vi "InitializeFpgaAcquisition.vi"(8 "error in (no error)":errorcluster, 11 "MCSA Acquisition Config":T1 {"FixedSizeX31"."InputConfig" items=["AC Coupled", "DC Coupled", "IEPE AC Coupled"]}) -> (0 "error out":errorcluster, 2 "start acquisition?":bool, 3 "dynamic FPGA VI reference":refnum<k20>)   [LabVIEW 2017, in "McsaFpgaAcquisition.lvlib"]
doc: "Initializes the acquisition of the dynamic channels with the RIO Wfm API."
uses:
  <vilib>/addons/InsightCM/Devices/Shared/Mcsa/McsaFpgaAcquisition/McsaFpgaAcquisition.lvlib
  <vilib>/addons/InsightCM/Devices/Shared/Mcsa/McsaFpgaAcquisition/controls/Configuration.ctl
  <vilib>/addons/InsightCM/Devices/Shared/Cms/CmsAcquisition/controls/FixedSizeArrays.ctl
  <vilib>/LabVIEW Targets/FPGA/cRIO/shared/nicrio_ModuleControls/nicrio_cRIO-9232_ConfigModeRing.ctl
  <vilib>/addons/InsightCM/Devices/Shared/Cms/cRIOWfmAcq/subVIs/RIO Wfm Cust Ctrls/rwfm_SamplingInfo.ctl
  <vilib>/addons/InsightCM/Devices/Shared/Mcsa/McsaFpgaAcquisition/controls/Group.ctl
  <vilib>/addons/InsightCM/Devices/Shared/Mcsa/McsaFpgaAcquisition/controls/ChannelMcsa.ctl
  <vilib>/addons/InsightCM/Devices/Shared/Mcsa/McsaFpgaAcquisition/controls/RangeParams.ctl
  <vilib>/Utility/error.llb/Error Cluster From Error Code.vi
  <vilib>/rvi/errors/niLvFpgaAdjustHostInterfaceError.vi
  <vilib>/rvi/interface/nirviReadWriteControl/nirviReadWriteControl.xnode
  <vilib>/addons/InsightCM/Devices/Shared/Mcsa/cRIOWfmAcqMcsa/cRIOWfmLibMcsa.lvlib
  NiFpgaLv.dll
  <vilib>/rvi/interface/Simulation/niFpgaSimulationCallBeginRW.vi
  <vilib>/addons/InsightCM/Devices/Shared/Cms/cRIOWfmAcq/cRIOWfmLib.lvlib
  <vilib>/addons/InsightCM/Devices/Shared/Cms/CmsAcquisition/CmsAcquisition.lvlib
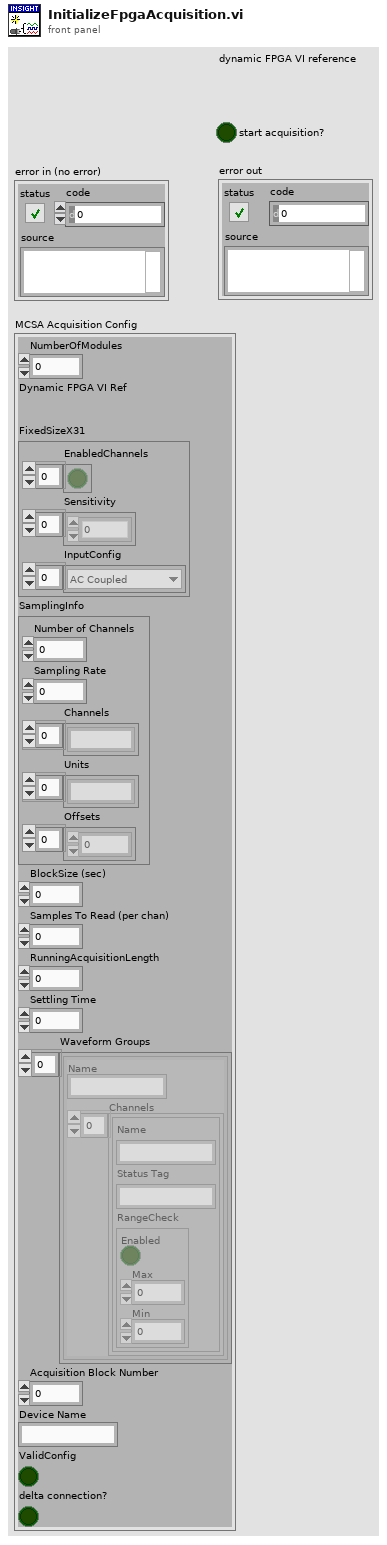
[diagram p1: front panel]
types:
  T1 = typedef "McsaFpgaAcquisition.lvlib/Configuration.ctl" = cluster{"NumberOfModules":i16, "Dynamic FPGA VI Ref":refnum<k20>, "FixedSizeX31":T2, "SamplingInfo":T4, "BlockSize (sec)":dbl, "Samples To Read (per chan)":i32, "RunningAcquisitionLength":dbl, "Settling Time":dbl, "Waveform Groups":T5[], "Acquisition Block Number":i32, "Device Name":string, "ValidConfig":bool, "delta connection?":bool}
  T2 = typedef "CmsAcquisition.lvlib/FixedSizeArrays.ctl" = cluster{"EnabledChannels":bool[], "Sensitivity":dbl[], "InputConfig":T3[]}
  T3 = typedef "nicrio_cRIO-9232_ConfigModeRing.ctl" = u8
  T4 = typedef "cRIOWfmLib.lvlib/rwfm_SamplingInfo.ctl" = cluster{"Number of Channels":i32, "Sampling Rate":dbl, "Channels":string[], "Units":string[], "Offsets":sgl[]}
  T5 = typedef "McsaFpgaAcquisition.lvlib/Group.ctl" = cluster{"Name":string, "Channels":T6[]}
  T6 = typedef "McsaFpgaAcquisition.lvlib/ChannelMcsa.ctl" = cluster{"Name":string, "Status Tag":string, "RangeCheck":T7}
  T7 = typedef "McsaFpgaAcquisition.lvlib/RangeParams.ctl" = cluster{"Enabled":bool, "Max":dbl, "Min":dbl}
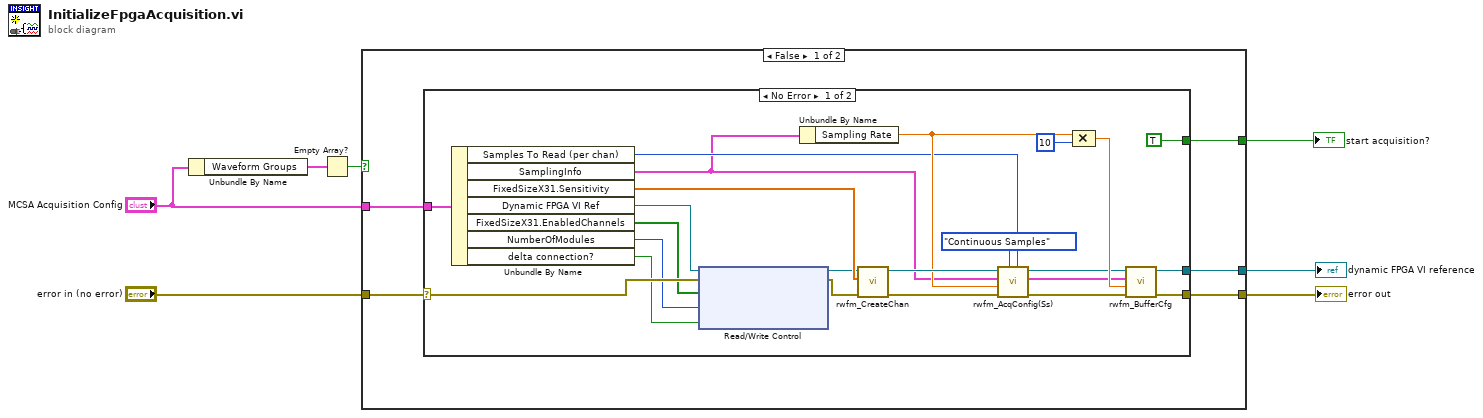
[diagram p0: block diagram]
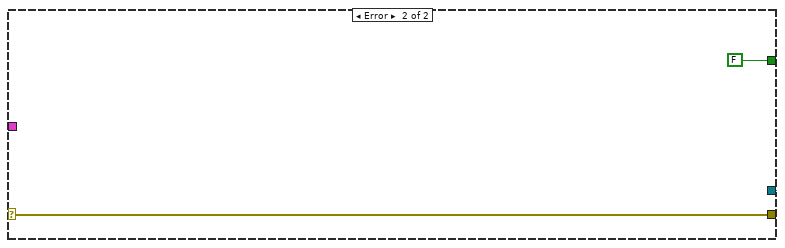
[diagram p2: hidden frame]
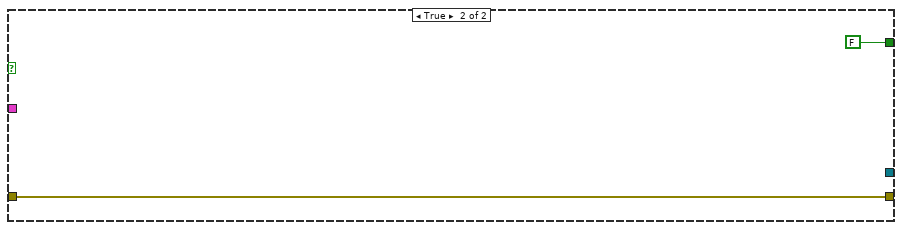
[diagram p3: hidden frame]
diagram:
  n1 = Unbundle By Name("MCSA Acquisition Config") -> ("Waveform Groups"=w4:T5[])
  n2 = Empty Array?(array=w4) -> (empty?=w2:bool)
  n3 = case shown="False" w2 {
    tunnel: "MCSA Acquisition Config" -> [w12 _]
    tunnel: [w11 w40] -> w7
    tunnel: "error in (no error)" -> [w10 w40]
    tunnel: [w9 _] -> w5
    tunnel: [w8 FALSE] -> w3
    frame False {
      n4 = case shown="No Error" w10 {
        selector: w10 -> [w31 w37]
        tunnel: w12 -> [w34 _]
        tunnel: [w33 w37] -> w11
        tunnel: [w32 refnum<k0> refnum] -> w9
        tunnel: [TRUE FALSE] -> w8
        frame No Error {
          n5 = Unbundle By Name(w34) -> ("Samples To Read (per chan)"=w18:i32, "SamplingInfo"=w15:T4, "FixedSizeX31.Sensitivity"=w35:dbl[], "Dynamic FPGA VI Ref"=w30:refnum<k20>, "FixedSizeX31.EnabledChannels"=w16:bool[], "NumberOfModules"=w17:i16, "delta connection?"=w13:bool)
          n6 = xnode "Read/Write Control"("FPGA VI Reference In"=w30, "error in"=w31, "Enable Chan Array"=w16, "Number of Modules"=w17, "delta connection? (F)"=w13) -> ("FPGA VI Reference Out"=w29:refnum<k20>, "error out"=w24:errorcluster)
          n7 = Unbundle By Name(w15) -> ("Sampling Rate"=w19:dbl)
          n8 = call <vilib>:"rwfm_CreateChan.vi"("error in"=w24, "Sensitivity"=w35, "Dynamic FPGA VI Reference"=w29) -> ("error out"=w20:errorcluster, "Dynamic FPGA VI Reference"=w21:refnum<k20>)  [unwired: 7 in]
          n9 = call <vilib>:"rwfm_AcqConfig(Ss).vi"("Samples per Channel"=w18, "Sample Mode"=enum16{"Finite Samples", "Continuous Samples"}."Continuous Samples", "error in"=w20, "Sample Rate S/s"=w19, "Sampling Info In"=w15, "Dynamic FPGA Ref"=w21) -> ("error out"=w22:errorcluster, "Sampling Info Out"=w26:T4, "Dynamic FPGA Ref Out"=w23:refnum<k20>)  [unwired: 2 in, 1 out]
          n10 = Compound Arithmetic op=MULTIPLY(w19, 10 ("value")) -> (w27:dbl)
          n11 = call <vilib>:"rwfm_BufferCfg.vi"("error in"=w22, "Buffer Size [Samps per Chan]"=w27, "Sampling Info In"=w26, "Dynamic FPGA VI Reference"=w23) -> ("error out"=w33:errorcluster, "Dynamic FPGA VI Reference"=w32:refnum<k20>)  [unwired: 4 in, 2 out]
        }
        frame Error {
          (unwired) cluster{"valid":bool, "description":string} {"valid"=FALSE, "description"=""} ("ConfigStatus")
        }
      }
    }
    frame True {
    }
  }
  "error out" <- w7
  "dynamic FPGA VI reference" <- w5
  "start acquisition?" <- w3
